vi "Power Control.vi"(6 "error in":errorcluster, 8 "Current":string="1", 9 "Voltage":string="4.5", 10 "Channel":enum16{"P6V", "P25V", "N25V"}(ring)=enum."P25V", 11 "command":T1(ring)) -> (0 "error out":errorcluster, 3 "Out":string)   [LabVIEW 2009]
uses:
  Global/Global 1.vi
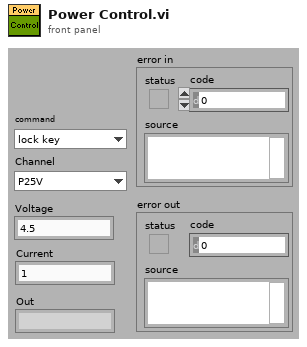
[diagram p1: front panel]
types:
  T1 = enum16{"lock key", "POwer OFF", "Power ON", "SET Volt and Current"}
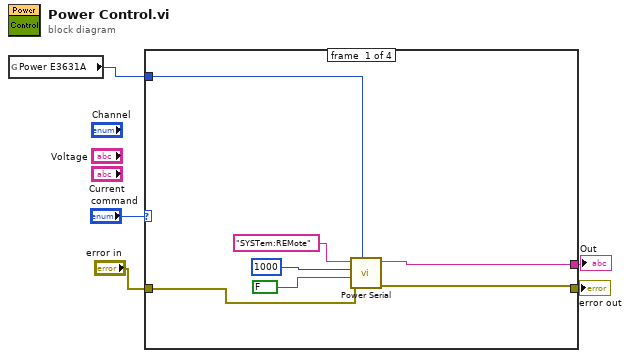
[diagram p0: block diagram]
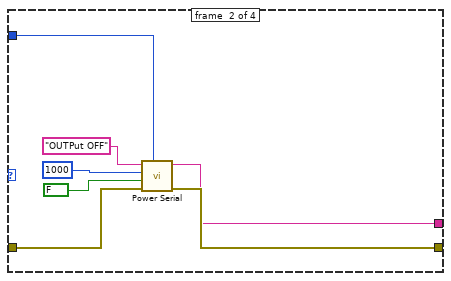
[diagram p2: hidden frame]
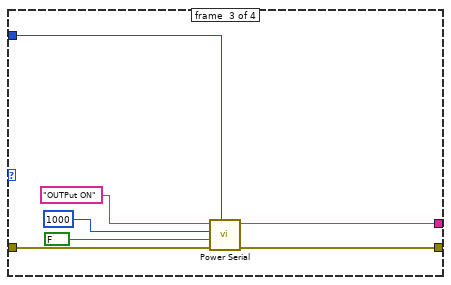
[diagram p3: hidden frame]
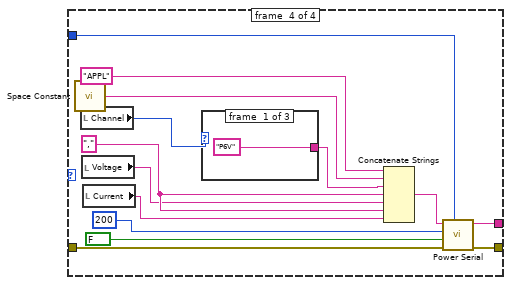
[diagram p4: hidden frame]
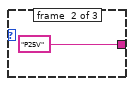
[diagram p5: hidden frame]
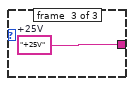
[diagram p6: hidden frame]
diagram:
  n1 = global read "Global 1.vi" "Power E3631A"() -> (w1:i32)
  n2 = case shown="\"SET Volt and Current\"" "command" {
    tunnel: w1 -> [w6 w16 w25 w40]
    tunnel: "error in" -> [w7 w15 w22 w37]
    tunnel: [w8 w14 w21 w36] -> w5
    tunnel: [w9 w13 w20 w35] -> w4
    frame #0 {
      n3 = call "Power Serial.vi"("VISA Resource Address"=w6, "error in (no error)"=w7, "Rd?"=FALSE, "Delay"=1000, "IN"="SYSTem:REMote" ("In")) -> ("error out"=w8:errorcluster, "OUT"=w9:string)  [unwired: 5 out]
    }
    frame #1 {
      n4 = call "Power Serial.vi"("VISA Resource Address"=w16, "error in (no error)"=w15, "Rd?"=FALSE, "Delay"=1000, "IN"="OUTPut OFF" ("In")) -> ("error out"=w14:errorcluster, "OUT"=w13:string)  [unwired: 5 out]
    }
    frame #2 {
      n5 = call "Power Serial.vi"("VISA Resource Address"=w25, "error in (no error)"=w22, "Rd?"=FALSE, "Delay"=1000, "IN"="OUTPut ON" ("In")) -> ("error out"=w21:errorcluster, "OUT"=w20:string)  [unwired: 5 out]
    }
    frame #3 {
      w32 = ","
      n6 = call <vilib>:"Space Constant.vi"() -> ("String"=w27:string)
      n7 = local read "Channel"() -> (w29:enum16{"P6V", "P25V", "N25V"})
      n8 = local read "Voltage"() -> (w31:string)
      n9 = local read "Current"() -> (w30:string)
      n10 = case shown="\"N25V\"" w29 {
        tunnel: ["P6V" "P25V" w43] -> w28
        frame #0 {
        }
        frame #1 {
        }
        frame #2 {
          w43 = "+25V"  # +25V
        }
      }
      n11 = Concatenate Strings("APPL" ("In"), w27, w28, w32, w31, w32, w30) -> (w34:string)
      n12 = call "Power Serial.vi"("VISA Resource Address"=w40, "error in (no error)"=w37, "Rd?"=FALSE, "Delay"=200, "IN"=w34) -> ("error out"=w36:errorcluster, "OUT"=w35:string)  [unwired: 5 out]
    }
  }
  "error out" <- w5
  "Out" <- w4
